vi "SAM to Tone.vi"(1 "SAM":T1) -> (0 "Tone":T2)   [LabVIEW 2015]
uses:
  Waveform VIs/Tone VIs/Tone Params.ctl
  SAM Params.ctl
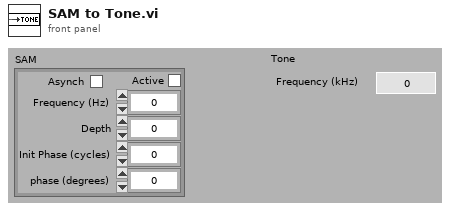
[diagram p1: front panel]
types:
  T1 = typedef "SAM Params.ctl" = cluster{"Active":bool, "Frequency (Hz)":dbl, "Depth":dbl, "Init Phase (cycles)":dbl, "phase (degrees)":dbl, "Asynch":bool}
  T2 = typedef "Tone Params.ctl" = cluster{"Frequency (kHz)":dbl, "Last Freq":dbl, "Last Phase":dbl}
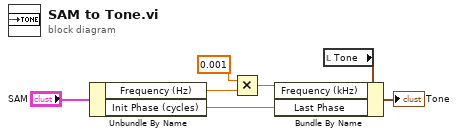
[diagram p0: block diagram]
diagram:
  n1 = Unbundle By Name("SAM") -> ("Frequency (Hz)"=w5:dbl, "Init Phase (cycles)"=w6:dbl)
  n2 = Multiply(x=0.001, y=w5) -> (x*y=w2:dbl)
  n3 = local read "Tone"() -> (w3:T2)
  n4 = Bundle By Name(cluster=w3, "Frequency (kHz)"=w2, "Last Phase"=w6) -> (→"Tone":T2)
